vi "dfd_Match Complex Zeros with Real Poles.vi"(10 "real poles":cdb[](array[numeric]), 11 "conj zeros":cdb[](array[numeric])) -> (1 "matched z&p":cluster{"zeros":cdb[], "poles":cdb[]}[](array[cluster]), 2 "remaining poles":cdb[](array[numeric]), 3 "remaining zeros":cdb[](array[numeric]))   [LabVIEW 2017, in "NI_DigFilterLicensed.lvlib"]
uses:
  <vilib>/addons/Digital Filter Design/NI_DigFilterLicensed.lvlib
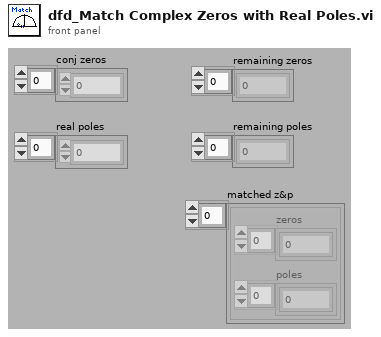
[diagram p1: front panel]
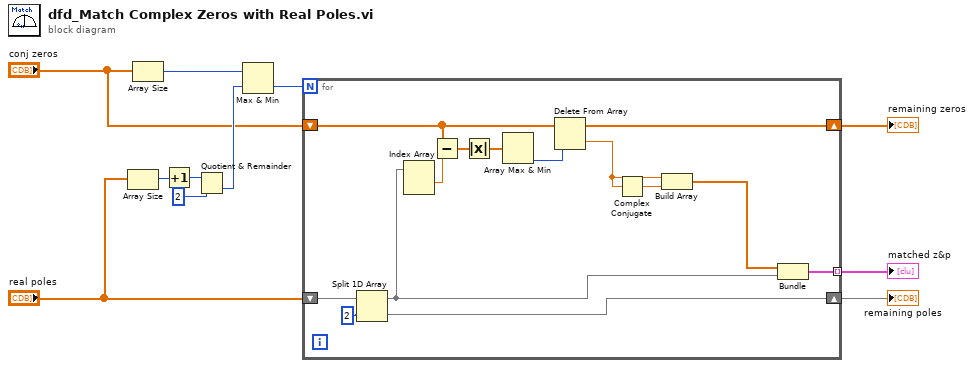
[diagram p0: block diagram]
diagram:
  n1 = Array Size(array="real poles") -> (size(s)=w6:i32)
  n2 = Array Size(array="conj zeros") -> (size(s)=w1:i32)
  n3 = Increment(x=w6) -> (x+1=w5:i32)
  n4 = Quotient & Remainder(x=w5, y=2) -> (floor(x/y)=w7:i32)  [unwired: 1 out]
  n5 = Max & Min(x=w1, y=w7) -> (min(x,y)=w8:i32)  [unwired: 1 out]
  n6 = for {
    N: w8 -> [_]
    shift-right: [w12] -> w11
    shift-left: "conj zeros" -> [w23]
    shift-right: [w20] -> w10
    shift-left: "real poles" -> [w22]
    tunnel: [w17] -> w2 mode=indexing
    n7 = Split 1D Array(array=w22, index=2) -> (first subarray=w18:cdb[], second subarray=w20:cdb[])
    n8 = Index Array(array=w18) -> (element #1=w19:cdb)  [unwired: 2 in, 1 out]
    n9 = Subtract(x=w23, y=w19) -> (x-y=w25:cdb[])
    n10 = Absolute Value(x=w25) -> (abs(x)=w24:dbl[])
    n11 = Array Max & Min(array=w24) -> (min index (indices)=w16:i32)  [unwired: 3 out]
    n12 = Delete From Array(array=w23, index=w16) -> (deleted portion=w14:cdb, array with subset deleted=w12:cdb[])  [unwired: 1 in]
    n13 = Complex Conjugate(1:w14) -> (0:w15:cdb)
    n14 = Build Array(w14, w15) -> (w13:cdb[])
    n15 = Bundle(w13, w18) -> (w17:cluster{cdb[], cdb[]})  [unwired: 1 out]
  }
  "remaining zeros" <- w11
  "remaining poles" <- w10
  "matched z&p" <- w2
